vi "Measure IV curves hysteresis sequence in same file 2420.vi"() -> ()   [LabVIEW 2014]
uses:
  Environmental Chamber LabVIEW and Instruments/Drivers and Software/LabVIEW 8.2 Drivers/keithley_24xx/Keithley 24XX/Public/Data/Read (Single Point).vi
  <vilib>/Utility/file.llb/Write To Spreadsheet File (string).vi
  Environmental Chamber LabVIEW and Instruments/Drivers and Software/keithley_24xx/Keithley 24XX/Keithley 24XX.lvlib
panel:
  in  "reverse?":bool
  in  "run!":bool
  out "Points to measure":dbl[](array[numeric])
  in  "voltage settings":T1={"+/-V"=-0.5, "steps"=100.0, "# of curves"=1, "Delay (min)"=0.02} {"Delay (min)" min=0.0 format="%#_13g"; "# of curves" step=1}
  out "File path":path
  in  "STOP":bool
  out "2420 IV curve":cluster{"X":dbl[], "Y":dbl[]}[](graph)
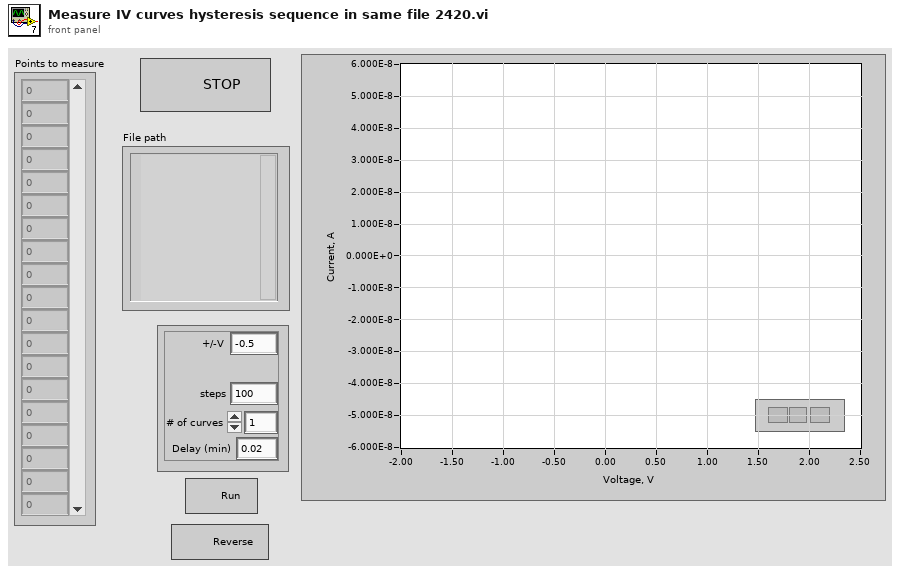
[diagram p1: front panel]
types:
  T1 = cluster{"+/-V":dbl, "steps":dbl, "# of curves":u32, "Delay (min)":dbl}
  T2 = enum16{"open", "open or create", "create or replace", "create", "open (read only)"}
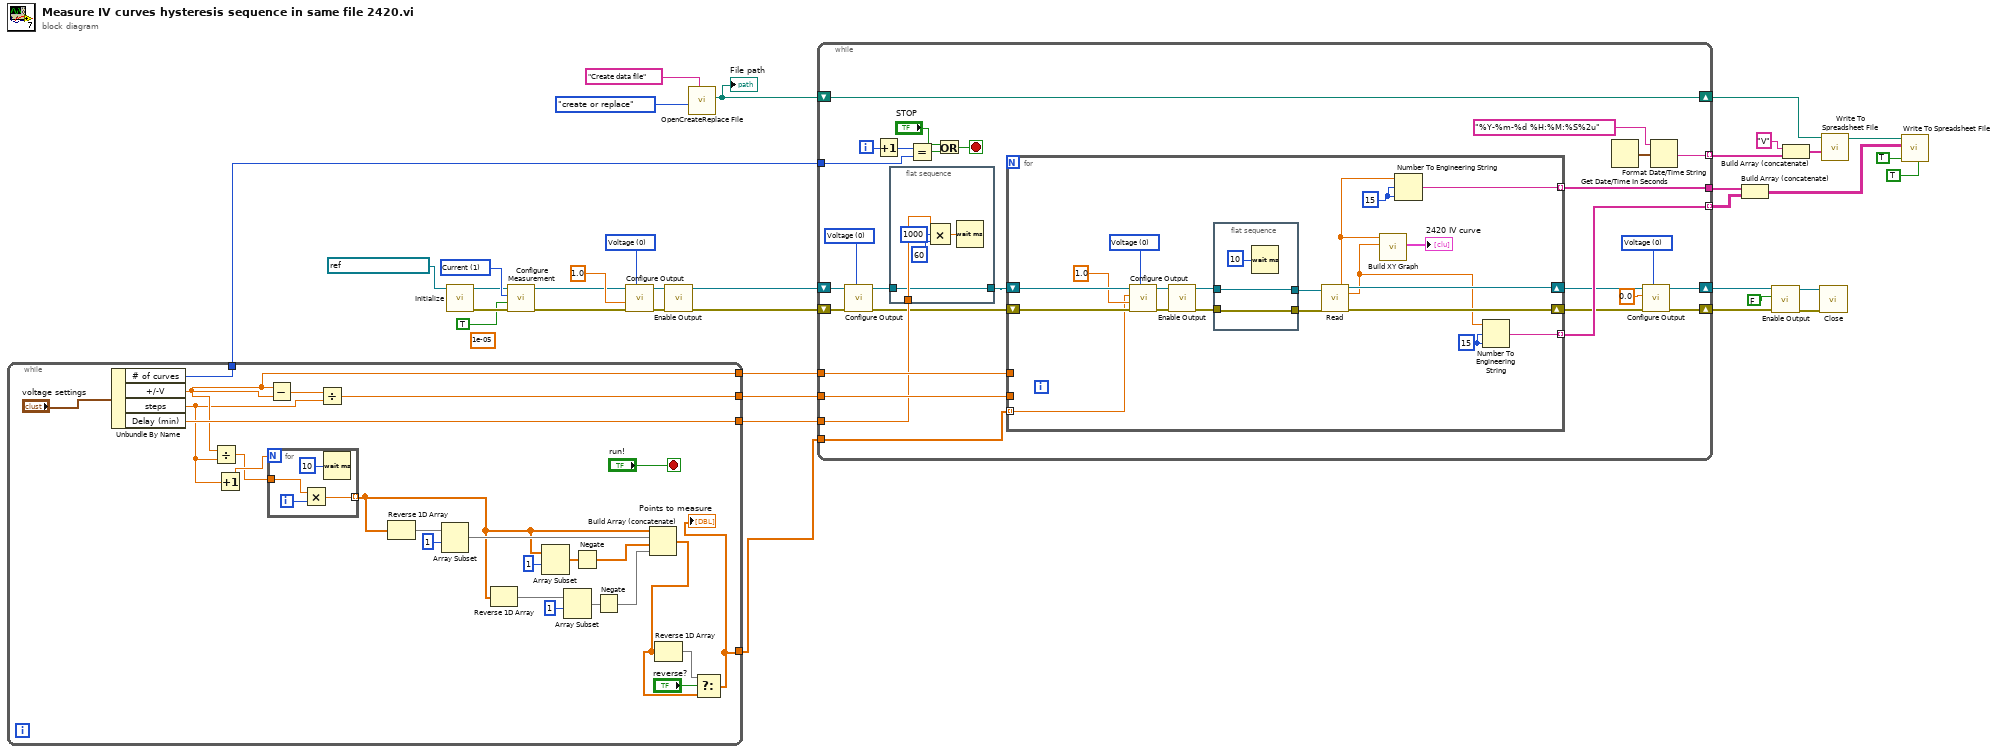
[diagram p0: block diagram]
diagram:
  w8 = u16 0 items=["Voltage", "Current"] ("Source Mode  (0: Voltage)")
  (unwired) 1e-05 ("Manual Range (1.0)")
  w34 = u16 1 items=["Volts", "Current", "Resistance"] ("Function (0: Volts)")
  n1 = while {
    tunnel: [w60] -> w36
    tunnel: [w58] -> w30
    tunnel: [w57] -> w29
    tunnel: [w51] -> w10
    tunnel: [w37] -> w1
    stop <- "run!" stop-if-true
    n2 = Unbundle By Name("voltage settings") -> ("# of curves"=w58:u32, "+/-V"=w51:dbl, "steps"=w50:dbl, "Delay (min)"=w57:dbl)
    n3 = Divide(x=w51, y=w50) -> (x/y=w55:dbl)
    n4 = Increment(x=w50) -> (x+1=w56:dbl)
    n5 = Subtract(x=w51, y=w51) -> (x-y=w61:dbl)
    n6 = for {
      N: w56 -> [_]
      tunnel: w55 -> [w65]
      tunnel: [w62] -> w42 mode=indexing
      i -> [w64]
      n7 = Multiply(x=w65, y=w64) -> (x*y=w62:dbl)
      n8 = Wait (ms)(milliseconds to wait=u32 10) -> ()  [unwired: 1 out]
    }
    n9 = Divide(x=w61, y=w50) -> (x/y=w60:dbl)
    n10 = Reverse 1D Array(array=w42) -> (reversed array=w53:dbl[])
    n11 = Array Subset(array=w53, index=1) -> (w48:dbl[])  [unwired: 1 in]
    n12 = Reverse 1D Array(array=w42) -> (reversed array=w44:dbl[])
    n13 = Array Subset(array=w42, index=1) -> (w41:dbl[])  [unwired: 1 in]
    n14 = Array Subset(array=w44, index=1) -> (w45:dbl[])  [unwired: 1 in]
    n15 = Negate(x=w41) -> (-x=w46:dbl[])
    n16 = Negate(x=w45) -> (-x=w43:dbl[])
    n17 = Build Array (concatenate)(w42, w48, w46, w43) -> (w38:dbl[])
    n18 = Reverse 1D Array(array=w38) -> (reversed array=w39:dbl[])
    n19 = Select(t=w39, s="reverse?", f=w38) -> (s? t:f=w37:dbl[])
    "Points to measure" <- w37
  }
  n20 = call "Initialize.vi"("VISA resource name"=refnum<visa-resource-name> "GPIB1::24::INSTR") -> ("error out"=w32:errorcluster, "VISA resource name out"=w33:refnum<visa-resource-name>)  [unwired: 9 in]
  n21 = call "Configure Measurement.vi"("error in (no error)"=w32, "Enable Auto Range (T:Enable)"=TRUE, "Function (0: Volts)"=w34, "VISA resource name"=w33) -> ("error out"=w3:errorcluster, "VISA resource name out"=w6:refnum<visa-resource-name>)  [unwired: 6 in]
  n22 = call "Configure Output.vi"("Source Mode  (0: Voltage)"=w8, "error in (no error)"=w3, "Compliance  Level (0.1)"=1.0, "VISA resource name"=w6) -> ("error out"=w4:errorcluster, "VISA resource name out"=w7:refnum<visa-resource-name>)  [unwired: 6 in]
  n23 = call "Enable Output.vi"("error in (no error)"=w4, "VISA resource name"=w7) -> ("error out"=w2:errorcluster, "VISA resource name out"=w5:refnum<visa-resource-name>)  [unwired: 8 in]
  n24 = call "OpenCreateReplace File.vi"("prompt"="Create data file", "function (open:0)"=T2."create or replace") -> ("new file path"=w26:path)  [unwired: 6 in, 3 out]
  "File path" <- w26
  n25 = while {
    tunnel: w10 -> [w93]
    tunnel: w36 -> [w92]
    shift-right: [w74] -> w21
    shift-left: w2 -> [w68]
    shift-right: [w76] -> w22
    shift-left: w5 -> [w70]
    shift-right: [w85] -> w19
    shift-left: w26 -> [w85]
    tunnel: w30 -> [w87]
    tunnel: w29 -> [w86]
    tunnel: [w82] -> w16 mode=indexing
    tunnel: [w81] -> w14
    tunnel: [w80] -> w13 mode=indexing
    tunnel: w1 -> [w66]
    i -> [w79]
    stop <- w91 stop-if-true
    w71 = u16 0 items=["Voltage", "Current"] ("Source Mode  (0: Voltage)")
    w78 = u16 0 items=["Voltage", "Current"] ("Source Mode  (0: Voltage)")
    n26 = call "Configure Output.vi"("Source Mode  (0: Voltage)"=w71, "error in (no error)"=w68, "VISA resource name"=w70) -> ("error out"=w67:errorcluster, "VISA resource name out"=w69:refnum<visa-resource-name>)  [unwired: 7 in]
    n27 = Increment(x=w79) -> (x+1=w89:i32)
    n28 = flat-sequence {
      tunnel: w69 -> [w117]
      tunnel: w86 -> [w118]
      tunnel: [w117] -> w72
      frame #0 {
        n29 = Compound Arithmetic op=MULTIPLY(w118, u32 1000 ("value"), u32 60 ("value")) -> (w121:dbl)
        n30 = Wait (ms)(milliseconds to wait=w121) -> ()  [unwired: 1 out]
      }
    }
    n31 = Equal?(x=w89, y=w87) -> (x = y?=w88:bool)
    n32 = Or(x="STOP", y=w88) -> (x .or. y?=w91:bool)
    n33 = for {
      tunnel: [w106] -> w80 mode=indexing
      shift-right: [w112] -> w75
      shift-left: w67 -> [w111]
      shift-right: [w113] -> w77
      shift-left: w72 -> [w110]
      tunnel: w92 -> [_]
      tunnel: w93 -> [_]
      tunnel: [w101] -> w81 mode=indexing
      tunnel: w66 -> [w94] mode=indexing
      w99 = i16 15 ("precision (6)")
      w100 = i16 15 ("precision (6)")
      w107 = u16 0 items=["Voltage", "Current"] ("Source Mode  (0: Voltage)")
      n34 = call "Configure Output.vi"("Source Mode  (0: Voltage)"=w107, "error in (no error)"=w111, "Compliance  Level (0.1)"=1.0, "Output Level (0)"=w94, "VISA resource name"=w110) -> ("error out"=w109:errorcluster, "VISA resource name out"=w108:refnum<visa-resource-name>)  [unwired: 5 in]
      n35 = call "Enable Output.vi"("error in (no error)"=w109, "VISA resource name"=w108) -> ("error out"=w102:errorcluster, "VISA resource name out"=w105:refnum<visa-resource-name>)  [unwired: 8 in]
      n36 = flat-sequence {
        tunnel: [w116] -> w104
        tunnel: w105 -> [w116]
        tunnel: w102 -> [w115]
        tunnel: [w115] -> w103
        frame #0 {
          n37 = Wait (ms)(milliseconds to wait=10 ("x")) -> ()  [unwired: 1 out]
        }
      }
      n38 = call-poly "Read.vi"("VISA resource name"=w104, "error in (no error)"=w103) -> ("Voltage"=w97:sgl, "VISA resource name out"=w113:refnum<visa-resource-name>, "Current"=w98:sgl, "error out"=w112:errorcluster)  [unwired: 7 in, 3 out]
      n39 = call "Build XY Graph"("Y Input"=w98, "X Input"=w97) -> ("XY Graph"=→"2420 IV curve":cluster{"X":dbl[], "Y":dbl[]}[])  [unwired: 8 in, 1 out]
      n40 = Number To Engineering String(2:w99, 3:w99, 4:w97) -> (0:w101:string)  [unwired: 1 in]
      n41 = Number To Engineering String(2:w100, 3:w100, 4:w98) -> (0:w106:string)  [unwired: 1 in]
    }
    n42 = Get Date/Time In Seconds() -> (seconds since 1Jan1904=w84:timestamp)
    n43 = call "Configure Output.vi"("Source Mode  (0: Voltage)"=w78, "error in (no error)"=w75, "Output Level (0)"=0.0, "VISA resource name"=w77) -> ("error out"=w74:errorcluster, "VISA resource name out"=w76:refnum<visa-resource-name>)  [unwired: 6 in]
    n44 = Format Date/Time String(time format string (%c)="%Y-%m-%d %H:%M:%S%2u", seconds (now)=w84) -> (date/time string=w82:string)  [unwired: 1 in]
  }
  n45 = Build Array (concatenate)(w14, w13) -> (w12:string[][])
  n46 = call "Enable Output.vi"("error in (no error)"=w21, "Enable Output (T: Enable)"=FALSE, "VISA resource name"=w22) -> ("error out"=w23:errorcluster, "VISA resource name out"=w25:refnum<visa-resource-name>)  [unwired: 7 in]
  n47 = Build Array (concatenate)("V", w16) -> (w15:string[])
  n48 = call "Close.vi"("error in (no error)"=w23, "VISA resource name"=w25) -> ()  [unwired: 9 in, 1 out]
  n49 = call-poly <vilib>:"Write To Spreadsheet File.vi"("1D data"=w15, "file path (dialog if empty)"=w19) -> ("new file path (Not A Path if cancelled)"=w18:path)  [unwired: 6 in]
  n50 = call-poly <vilib>:"Write To Spreadsheet File.vi"("transpose? (no:F)"=TRUE, "append to file? (new file:F)"=TRUE ("transpose? (no:F)"), "2D data"=w12, "file path (dialog if empty)"=w18) -> ()  [unwired: 4 in, 1 out]
